vi "FPGA_DAQ_Int.vi"() -> ()   [LabVIEW 2019]
doc: "This VI provides a template for customizing a waveform acquisition using delta-sigma based NI C Series analog input smodules."
uses:
  <vilib>/LabVIEW Targets/FPGA/cRIO/shared/nicrio_ModuleControls/nicrio_cRIO-9219_ConversionTime.ctl
  <vilib>/rvi/Emulation/niFpgaSctlEmulationGetInTimedLoop.vi
  <vilib>/rvi/Emulation/niFpgaProcessEmulError.vi
  <vilib>/LabVIEW Targets/FPGA/cRIO/shared/nicrio_DsaDataRateApi/_nicrio_9234GetDataRate131.vi
  <vilib>/LabVIEW Targets/FPGA/cRIO/shared/nicrio_DsaDataRateApi/_nicrio_9225GetDataRate131.vi
  <vilib>/rvi/eio/common/nirviEmuTemplatePropertySet_errors.vi
  <vilib>/rvi/eio/common/nirviEmuTemplatePropertyGet_noerrors.vi
  <vilib>/rvi/eio/common/nirviEmuTemplateMethod_errors.vi
  <vilib>/rvi/Emulation/niFpgaGetClockAttributes.vi
  <vilib>/rvi/Emulation/niFpgaEmulationReportErrorSimple.vi
  <vilib>/rvi/Emulation/niFpgaCriticalErrorInLSC.vi
  <vilib>/rvi/interface/RandomDataEmulation/niFpgaRandomDataHandleErrors.vi
  <vilib>/eio/EIOPropertyNode/EIOPropertyNode.xnode
  <vilib>/LabVIEW Targets/FPGA/cRIO/shared/nicrio_ModuleControls/nicrio_cRIO-9234_DataRatesRing2.ctl
  <vilib>/LabVIEW Targets/FPGA/cRIO/shared/nicrio_ModuleControls/nicrio_cRIO-9225_DataRatesRing.ctl
  <vilib>/eio/EIONode/EIONode.xnode
  <vilib>/rvi/DataTransferAndStorage/Container/XNode/niFpgaContainer.xnode
  <vilib>/rvi/interface/RandomDataEmulation/nirviRandomDataFpgaReadWriteTemplate.vi
  <vilib>/rvi/eio/common/nirviEmuTemplatePropertyGet_errors.vi
  <vilib>/rvi/eio/common/nirviEmuTemplatePropertySet_noerrors.vi
panel:
  in  "stop":bool
  out "Temp0 D2":u32
  out "Temp1 D2":u32
  out "Temp2 D2":u32
  out "Temp3 D2":u32
  out "Calibration Voltage (NI 9225)":cluster{"LSB Weight":u32, "Offset":i32}[](array[cluster])
  out "Calibration Vibration (NI 9234)":cluster{"LSB Weight":u32, "Offset":i32}[](array[cluster])
  out "Calibration Current (NI 9215)":cluster{"LSB Weight":u32, "Offset":i32}[](array[cluster])
  out "error out":errorcluster
  in  "Measurements per cycle":i16=25600
  out "StopGeral":bool
  out "CJC1":u32
  out "CJC0":u32
  out "Temp3":u32
  out "Temp2":u32
  out "Temp1":i32
  out "Temp0":i32
  out "Acq Loop uS":u32
  out "FPGA Error":errorcluster
  out "Module Underflow":bool
  out "Finished":bool
  out "First Read":bool
  out "DMA FIFO Full":bool
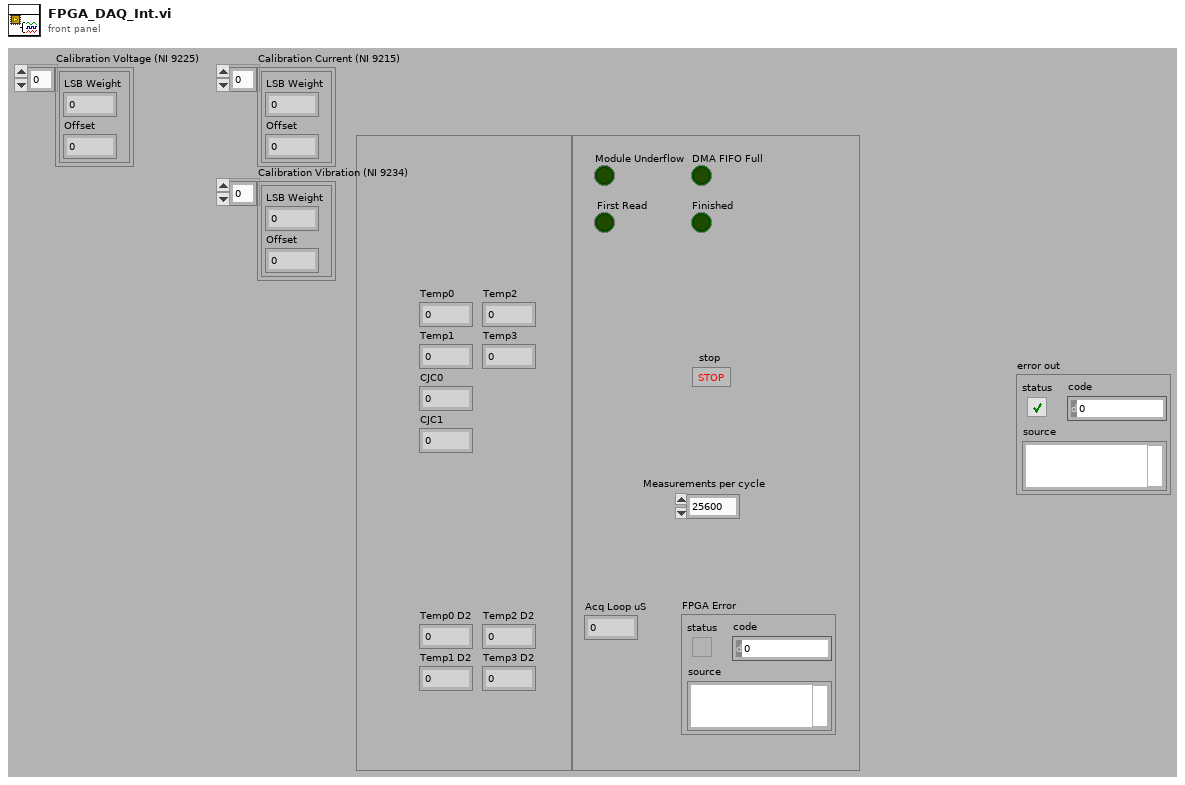
[diagram p1: front panel]
types:
  T1 = typedef "nicrio_cRIO-9219_ConversionTime.ctl" = enum8{"High Speed", "Best 60 Hz Rejection", "Best 50 Hz Rejection", "High Resolution"}
  T2 = typedef "nicrio_cRIO-9225_DataRatesRing2.ctl" = u8
  T3 = typedef "nicrio_cRIO-9234_DataRatesRing2.ctl" = u8
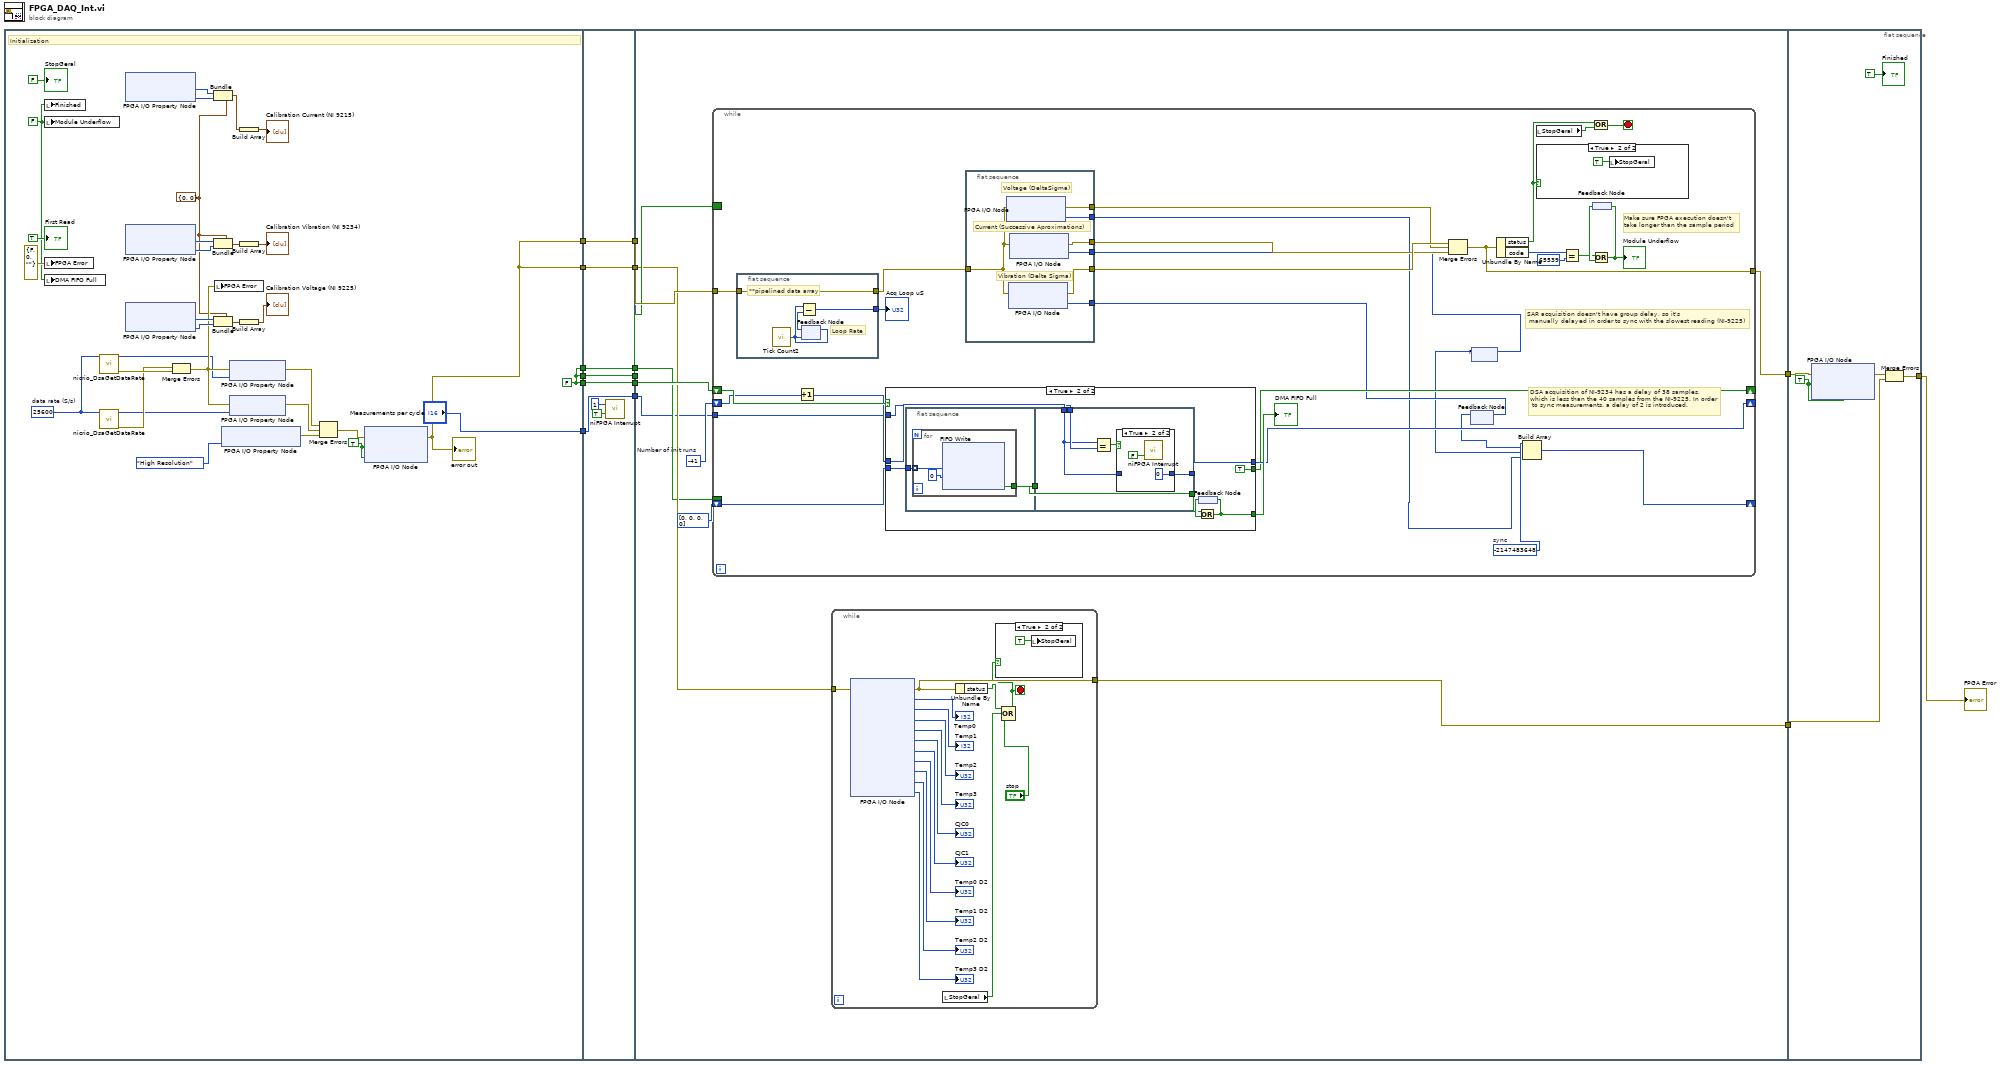
[diagram p0: block diagram]
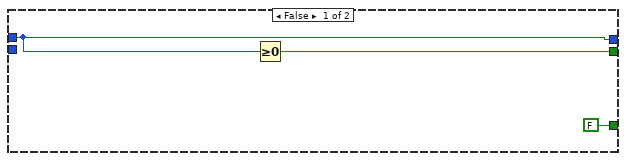
[diagram p4: hidden frame]
diagram:
  n1 = flat-sequence {
    tunnel: [w46] -> w14
    tunnel: [w47] -> w13
    tunnel: [w47] -> w12
    tunnel: [w47] -> w11
    tunnel: [w46] -> w10
    tunnel: ["Measurements per cycle"] -> w9
    tunnel: w14 -> [w55]
    tunnel: [w55] -> w8
    tunnel: w13 -> [w54]
    tunnel: [w54] -> w7
    tunnel: w12 -> [w53]
    tunnel: [w53] -> w6
    tunnel: w11 -> [w52]
    tunnel: [w52] -> w5
    tunnel: w10 -> [w51]
    tunnel: [w51] -> w4
    tunnel: w9 -> [w50]
    tunnel: [w50] -> w3
    tunnel: w8 -> [w65]
    tunnel: [w63] -> w2
    tunnel: w7 -> [w59]
    tunnel: w6 -> [w62]
    tunnel: w5 -> [w64]
    tunnel: w4 -> [w61]
    tunnel: [w60] -> w1
    tunnel: w3 -> [w57]
    tunnel: w2 -> [w153]
    tunnel: [w151] -> w15
    tunnel: w1 -> [w150]
    frame #0 {
      w31 = u32 25600  # data rate (S/s)
      w20 = cluster{"LSB Weight":u32, "Offset":i32} {"LSB Weight"=0, "Offset"=0}
      w41 = FALSE ("Module Underflow")
      w42 = TRUE ("Mod1/Start")
      w47 = FALSE
      # "Initialization"
      n2 = local write "Finished"(w41) -> ()
      n3 = local write "Module Underflow"(w41) -> ()
      n4 = local write "FPGA Error"(errorcluster {"status"=FALSE, "code"=0, "source"=""} ("FPGA Error")) -> ()
      n5 = local write "DMA FIFO Full"(w41) -> ()
      n6 = call-poly <vilib>:"nicrio_DsaGetDataRate.vi"("data rate (S/s)"=w31) -> ("data rate"=w28:T2, "error out"=w33:errorcluster)  [unwired: 10 in, 3 out]
      n7 = call-poly <vilib>:"nicrio_DsaGetDataRate.vi"("data rate (S/s)"=w31) -> ("data rate"=w27:T3, "error out"=w32:errorcluster)  [unwired: 10 in, 3 out]
      n8 = xnode "FPGA I/O Property Node"() -> ("LSB Weight"=w26:u32, "Offset"=w36:i32)  [unwired: 1 in, 1 out]
      n9 = xnode "FPGA I/O Property Node"() -> ("LSB Weight"=w23:u32, "Offset"=w24:i32)  [unwired: 1 in, 1 out]
      n10 = xnode "FPGA I/O Property Node"() -> ("LSB Weight"=w35:u32, "Offset"=w34:i32)  [unwired: 1 in, 1 out]
      n11 = Merge Errors(w32, w33) -> (w29:errorcluster)
      n12 = Bundle(cluster=w20, "LSB Weight"=w26, "Offset"=w36) -> (w22:cluster{"LSB Weight":u32, "Offset":i32})
      n13 = Bundle(cluster=w20, "LSB Weight"=w23, "Offset"=w24) -> (w19:cluster{"LSB Weight":u32, "Offset":i32})
      n14 = Bundle(cluster=w20, "LSB Weight"=w35, "Offset"=w34) -> (w17:cluster{"LSB Weight":u32, "Offset":i32})
      n15 = local write "FPGA Error"(w29) -> ()
      n16 = xnode "FPGA I/O Property Node"("Conversion Time"=nicrio_cRIO-9219_ConversionTime."High Resolution") -> ("error out"=w25:errorcluster)  [unwired: 2 in, 1 out]
      n17 = xnode "FPGA I/O Property Node"("error in"=w29, "Data Rate"=w28) -> ("error out"=w39:errorcluster)  [unwired: 1 in, 1 out]
      n18 = xnode "FPGA I/O Property Node"("error in"=w29, "Data Rate"=w27) -> ("error out"=w40:errorcluster)  [unwired: 1 in, 1 out]
      n19 = Build Array(w22) -> (→"Calibration Current (NI 9215)":cluster{"LSB Weight":u32, "Offset":i32}[])
      n20 = Build Array(w19) -> (→"Calibration Vibration (NI 9234)":cluster{"LSB Weight":u32, "Offset":i32}[])
      n21 = Build Array(w17) -> (→"Calibration Voltage (NI 9225)":cluster{"LSB Weight":u32, "Offset":i32}[])
      n22 = Merge Errors(w39, w40, w25) -> (w38:errorcluster)
      n23 = xnode "FPGA I/O Node"("error in"=w38, "Mod3/Start"=w42, "Mod4/Start"=w42) -> ("error out"=w46:errorcluster)  [unwired: 2 in, 2 out]
      "error out" <- w46
      "First Read" <- TRUE ("First Read")
      "StopGeral" <- FALSE ("StopGeral")
    }
    frame #1 {
      n24 = call <vilib>:"niFPGA Interrupt.vi"("Wait Until Cleared (F)"=TRUE, "IRQ Number (0)"=u8 1) -> ()  [unwired: 1 in]
    }
    frame #2 {
      w58 = i16 -41  # Number of init runs
      n25 = while {
        tunnel: w65 -> [w110]
        tunnel: [w100] -> w63
        shift-right: [w89] -> _
        shift-left: w64 -> [w108]
        border: w59 -> [_]
        border: w62 -> [_]
        shift-right: [w91] -> _
        shift-left: i32[] [0, 0, 0, 0] -> [w90]
        shift-right: [w92] -> _
        shift-left: w58 -> [w95]
        tunnel: w57 -> [w93]
        stop <- w98 stop-if-true
        w88 = -2147483648  # sync
        # "DSA acquisition of NI-9234 has a delay of 38 samples,\nwhich is less than the 40 samples from the NI-9225. In order\n to sync measurements, a delay of 2 is introduced."
        # "SAR acquisition doesn't have group delay, so it's\n manually delayed in order to sync with the slowest reading (NI-9225)"
        # "Make sure FPGA execution doesn't\ntake longer than the sample period"
        n26 = flat-sequence {
          tunnel: [w149] -> w101
          tunnel: w110 -> [w149]
          tunnel: [w146] -> w109
          frame #0 {
            # "**pipelined data array"
            # "Loop Rate"
            n27 = call "Tick Count2"() -> ("Tick Count(uSec)"=w148:u32)
            n28 = feedback-in #1(w148) -> ()
            n29 = feedback #1(w148) -> (w147:u32)
            n30 = Subtract(x=w148, y=w147) -> (x-y=w146:u32)
          }
        }
        n31 = Increment(x=w95) -> (x+1=w94:i16)
        n32 = case shown="True" w108 {
          tunnel: [FALSE w126] -> w96
          tunnel: w94 -> [w122 w129]
          tunnel: w93 -> [_ w128]
          tunnel: [w122 w127] -> w92
          tunnel: w90 -> [_ w125]
          tunnel: [w121 TRUE] -> w89
          frame False {
            n33 = Greater Or Equal To 0?(x=w122) -> (x >= 0?=w121:bool)
          }
          frame True {
            n34 = flat-sequence {
              tunnel: [w134] -> w130
              tunnel: w125 -> [w133]
              tunnel: [w142] -> w131
              tunnel: w130 -> [w142]
              tunnel: w129 -> [w139]
              tunnel: w128 -> [w141]
              tunnel: [w138] -> w127
              frame #0 {
                n35 = for {
                  tunnel: [w137] -> w134
                  tunnel: w133 -> [w135] mode=indexing
                  n36 = xnode ("FIFO Write")("Element"=w135, "Timeout"=0) -> ("Timed Out?"=w137:bool)  [unwired: 1 in, 1 out]
                }
              }
              frame #1 {
                n37 = Equal?(x=w139, y=w141) -> (x = y?=w140:bool)
                n38 = case shown="True" w140 {
                  tunnel: w139 -> [w143 _]
                  tunnel: [w143 i16 0] -> w138
                  frame False {
                  }
                  frame True {
                    n39 = call <vilib>:"niFPGA Interrupt.vi"("Wait Until Cleared (F)"=FALSE) -> ()  [unwired: 2 in]
                  }
                }
              }
            }
            n40 = feedback #2() -> (w132:bool)
            n41 = Or(x=w131, y=w132) -> (x .or. y?=w126:bool)
            n42 = feedback-in #2(w126) -> ()
          }
        }
        "DMA FIFO Full" <- w96
        n43 = flat-sequence {
          tunnel: [w119] -> w104
          tunnel: [w118] -> w103
          tunnel: [w117] -> w102
          tunnel: w101 -> [w116]
          tunnel: [w115] -> w83
          tunnel: [w114] -> w87
          tunnel: [w113] -> w86
          frame #0 {
            # "Voltage (DeltaSigma)"
            # "Current (Successive Aproximations)"
            # "Vibration (Delta Sigma)"
            n44 = xnode "FPGA I/O Node"("error in"=w116) -> ("error out"=w118:errorcluster, "Mod4/AI0"=w115:i32)  [unwired: 1 in, 1 out]
            n45 = xnode "FPGA I/O Node"("error in"=w116) -> ("error out"=w119:errorcluster, "Mod3/AI1"=w113:i32)  [unwired: 1 in, 1 out]
            n46 = xnode "FPGA I/O Node"("error in"=w116) -> ("error out"=w117:errorcluster, "Mod2/AI3"=w114:i16)  [unwired: 1 in, 1 out]
          }
        }
        n47 = Merge Errors(w104, w103, w102) -> (w100:errorcluster)
        n48 = feedback #3() -> (w85:i32)  [unwired: 1 in]
        n49 = feedback-in #3(w86) -> ()
        n50 = feedback #4() -> (w84:i16)  [unwired: 1 in]
        n51 = feedback-in #4(w87) -> ()
        n52 = Unbundle By Name(w100) -> ("status"=w97:bool, "code"=w111:i32)
        n53 = Build Array(w88, w85, w84, w83) -> (w91:i32[])
        n54 = local read "StopGeral"() -> (w99:bool)
        n55 = case shown="True" w97 {
          frame False {
          }
          frame True {
            n56 = local write "StopGeral"(TRUE ("StopGeral")) -> ()
          }
        }
        n57 = Equal?(x=w111, y=65539) -> (x = y?=w106:bool)
        n58 = Or(x=w97, y=w99) -> (x .or. y?=w98:bool)
        n59 = feedback #5() -> (w107:bool)
        n60 = Or(x=w106, y=w107) -> (x .or. y?=w105:bool)
        "Module Underflow" <- w105
        n61 = feedback-in #5(w105) -> ()
        "Acq Loop uS" <- w109
      }
      n62 = while {
        tunnel: w61 -> [w75]
        tunnel: [w74] -> w60
        stop <- w66 stop-if-true
        n63 = xnode "FPGA I/O Node"("error in"=w75) -> ("error out"=w74:errorcluster, "Mod1/CH0"=→"Temp0":i32, "Mod1/CH1"=→"Temp1":i32, "Mod1/CH2"=→"Temp2":u32, "Mod1/CH3"=→"Temp3":u32, "Mod1/CJC0"=→"CJC0":u32, "Mod1/CJC1"=→"CJC1":u32, "Mod5/CH0"=→"Temp0 D2":u32, "Mod5/CH1"=→"Temp1 D2":u32, "Mod5/CH2"=→"Temp2 D2":u32, "Mod5/CH3"=→"Temp3 D2":u32)  [unwired: 10 in, 10 out]
        n64 = local read "StopGeral"() -> (w68:bool)
        n65 = Unbundle By Name(w74) -> ("status"=w69:bool)
        n66 = Compound Arithmetic op=OR(w69, w68, "stop") -> (w66:bool)
        n67 = case shown="True" w66 {
          frame False {
          }
          frame True {
            n68 = local write "StopGeral"(TRUE ("StopGeral")) -> ()
          }
        }
      }
    }
    frame #3 {
      w154 = TRUE ("Mod1/Stop")
      n69 = xnode "FPGA I/O Node"("error in"=w153, "Mod3/Stop"=w154, "Mod4/Stop"=w154) -> ("error out"=w152:errorcluster)  [unwired: 2 in, 2 out]
      n70 = Merge Errors(w152, w150) -> (w151:errorcluster)
      "Finished" <- TRUE ("Finished")
    }
  }
  "FPGA Error" <- w15
